vi "arc.vi"() -> ()   [LabVIEW 2018]
uses:
  <vilib>/MediaMongrels Ltd/WebSockets/WebSockets/WebSocket Client/WebSocket Client.lvclass
  D:/software_setup/National Instruments/LabVIEW 2018/vi.lib/MediaMongrels Ltd/WebSockets/WebSockets/WebSocket/WebSocket.lvclass
panel:
  in  "SetCircleCmd_toPoint":dbl[](array[numeric])
  in  "SetCircleCmd_cirPoint":dbl[](array[numeric])
  in  "count":dbl
  in  "SetARCCmd_toPoint":dbl[](array[numeric])
  in  "SetARCCmd_cirPoint":dbl[](array[numeric])
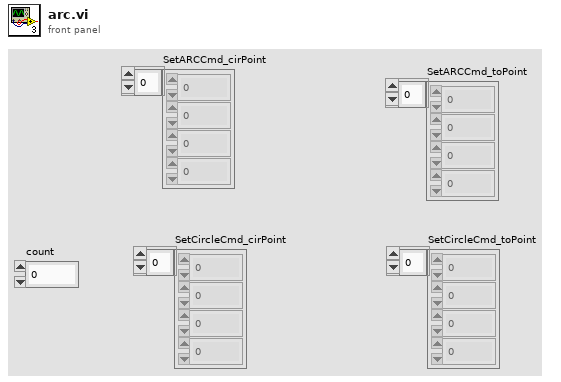
[diagram p1: front panel]
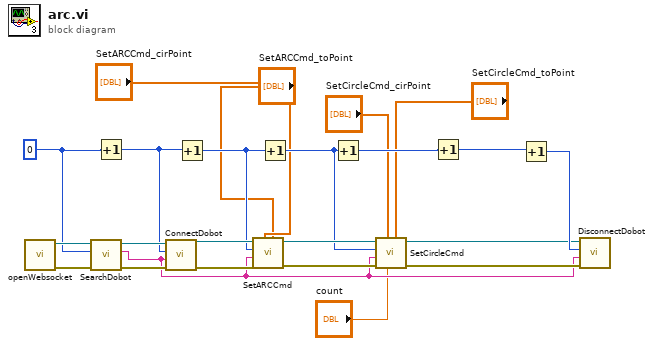
[diagram p0: block diagram]
diagram:
  w19 = 0 ("id")
  n1 = call <vilib>:"openWebsocket.vi"() -> ("error out"=w21:errorcluster, "WebSocket Client out"=w23:refnum<class "WebSocket Client.lvclass">)  [unwired: 10 in]
  n2 = call <vilib>:"SearchDobot.vi"("error in (no error)"=w21, "id"=w19, "WebSocket in"=w23) -> ("error out"=w20:errorcluster, "portName"=w6:string, "WebSocket out"=w22:refnum<class "WebSocket Client.lvclass">)  [unwired: 6 in]
  n3 = Increment(x=w19) -> (x+1=w18:i32)
  n4 = call <vilib>:"ConnectDobot.vi"("error in (no error)"=w20, "portName"=w6, "id"=w18, "WebSocket in"=w22) -> ("error out"=w9:errorcluster, "WebSocket out"=w14:refnum<class "WebSocket Client.lvclass">)  [unwired: 5 in, 1 out]
  n5 = Increment(x=w18) -> (x+1=w8:i32)
  n6 = call <vilib>:"SetARCCmd.vi"("toPoint"="SetARCCmd_toPoint", "cirPoint"="SetARCCmd_cirPoint", "error in (no error)"=w9, "portName"=w6, "id"=w8, "WebSocket in"=w14) -> ("error out"=w11:errorcluster, "WebSocket out"=w13:refnum<class "WebSocket Client.lvclass">)  [unwired: 3 in, 1 out]
  n7 = Increment(x=w8) -> (x+1=w7:i32)
  n8 = Increment(x=w7) -> (x+1=w16:i32)
  n9 = call <vilib>:"SetCircleCmd.vi"("toPoint"="SetCircleCmd_toPoint", "count"="count", "cirPoint"="SetCircleCmd_cirPoint", "error in (no error)"=w11, "portName"=w6, "id"=w7, "WebSocket in"=w13) -> ("error out"=w10:errorcluster, "WebSocket out"=w12:refnum<class "WebSocket Client.lvclass">)  [unwired: 2 in, 1 out]
  n10 = Increment(x=w16) -> (x+1=w15:i32)
  n11 = Increment(x=w15) -> (x+1=w17:i32)
  n12 = call <vilib>:"DisconnectDobot.vi"("error in (no error)"=w10, "portName"=w6, "id"=w17, "WebSocket in"=w12) -> ()  [unwired: 5 in, 3 out]
